vi "Create Antinode R-C.vi"(10 "2":i32, 11 "1":i32) -> (2 "Antinode 2":i32, 3 "Antinode 1":i32)   [LabVIEW 2024]
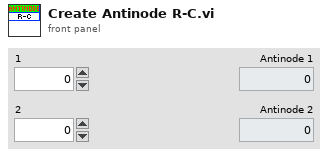
[diagram p1: front panel]
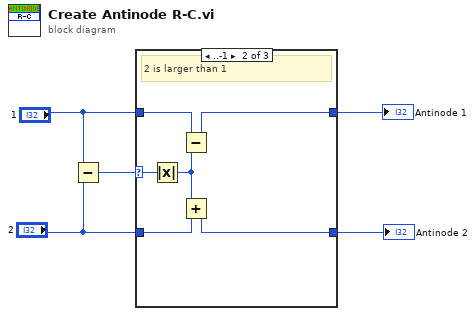
[diagram p0: block diagram]
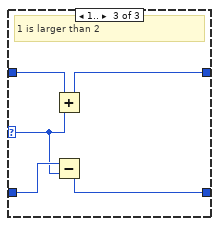
[diagram p3: hidden frame]
diagram:
  n1 = Subtract(x="1", y="2") -> (x-y=w5:i32)
  n2 = case shown="..-1" w5 {
    selector: w5 -> [_ w13 w16]
    tunnel: "1" -> [w6 w12 w17]
    tunnel: "2" -> [w7 w8 w18]
    tunnel: [w6 w10 w15] -> w2
    tunnel: [w7 w9 w14] -> w1
    frame 0 {
      # "Same"
    }
    frame ..-1 {
      # "2 is larger than 1"
      n3 = Absolute Value(x=w13) -> (abs(x)=w11:i32)
      n4 = Subtract(x=w12, y=w11) -> (x-y=w10:i32)
      n5 = Add(x=w11, y=w8) -> (x+y=w9:i32)
    }
    frame 1.. {
      # "1 is larger than 2"
      n6 = Add(x=w17, y=w16) -> (x+y=w15:i32)
      n7 = Subtract(x=w18, y=w16) -> (x-y=w14:i32)
    }
  }
  "Antinode 1" <- w2
  "Antinode 2" <- w1
